vi "SpaceAvailable.vi"(3 "error in (no error)":errorcluster, 5 "task in":refnum<k24>) -> (0 "error out":errorcluster, 1 "SpaceAvailable":u32, 2 "task out":refnum<k24>)   [LabVIEW 2010]
uses:
  C:/Program Files/National Instruments/LabVIEW 2010/vi.lib/ULx/ULx_LV.dll
  Program Files/National Instruments/LabVIEW 2010/vi.lib/ULx/ULx_LV.dll
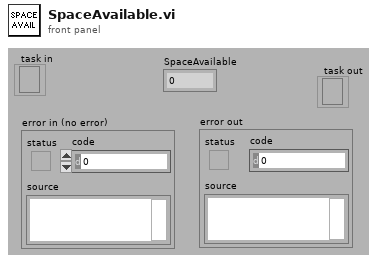
[diagram p1: front panel]
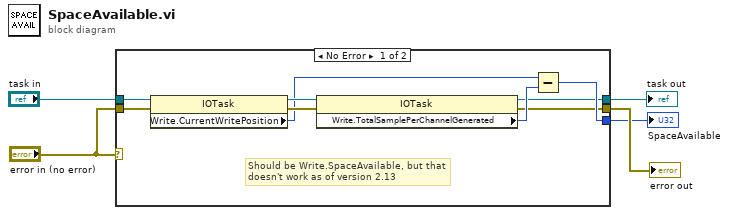
[diagram p0: block diagram]
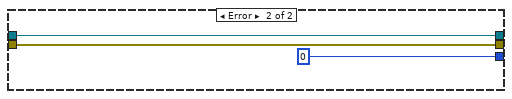
[diagram p2: hidden frame]
diagram:
  n1 = case shown="No Error" "error in (no error)" {
    tunnel: "task in" -> [w14 w17]
    tunnel: "error in (no error)" -> [w13 w16]
    tunnel: [w6 w17] -> w4
    tunnel: [w7 w16] -> w3
    tunnel: [w8 u32 0 ("Read.AvailableSamplePerChannel")] -> w1
    frame No Error {
      # "Should be Write.SpaceAvailable, but that \ndoesn't work as of version 2.13"
      n2 = property class="IOTask"(reference=w14, error in=w13) -> (reference out=w11:refnum<k24>, error out=w12:errorcluster, "Write.CurrentWritePosition"=w10:u32)
      n3 = property class="IOTask"(reference=w11, error in=w12) -> (reference out=w6:refnum<k24>, error out=w7:errorcluster, "Write.TotalSamplePerChannelGenerated"=w9:u32)
      n4 = Subtract(x=w10, y=w9) -> (x-y=w8:u32)
    }
    frame Error {
    }
  }
  "task out" <- w4
  "error out" <- w3
  "SpaceAvailable" <- w1
